vi "T0-T90.vi"(8 "error in (no error)":errorcluster caption="Fehler (Eingang, kein Fehler)", 9 "Umschaltzeitpunkte":timestamp[](array[timestamp]), 11 "T0-T90":timestamp[](array[timestamp])) -> (0 "error out":errorcluster caption="Fehler (Ausgang)", 1 "T100-T10":dbl[](array[numeric]), 3 "T0-T90":dbl[](array[numeric]))   [LabVIEW 2020, in "EPA 1065.lvlib" / "T90 Test 1065-308.lvlib"]
uses:
  T90 Test 1065-308.lvlib
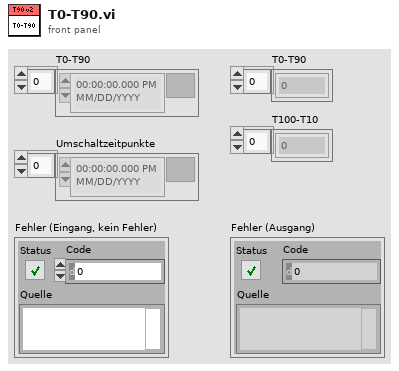
[diagram p1: front panel]
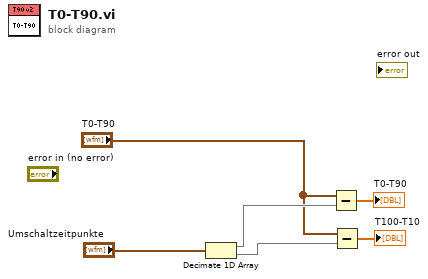
[diagram p0: block diagram]
diagram:
  n1 = Decimate 1D Array("Umschaltzeitpunkte") -> (w5:timestamp[], w4:timestamp[])
  n2 = Subtract(x="T0-T90", y=w5) -> (x-y=→"T0-T90":dbl[])
  n3 = Subtract(x="T0-T90", y=w4) -> (x-y=→"T100-T10":dbl[])
